vi "Get Conact Check State.vi"(8 "error in (no error)":errorcluster, 10 "Connections  (0: ANY)":u16(ring) items=["ANY", "ALL"], 11 "VISA resource name":refnum<visa-resource-name>="USB0::0x05E6::0x2461::04090176::INSTR") -> (0 "error out":errorcluster, 1 "Guard Check Pass":bool, 2 "Low Check Pass":bool, 3 "VISA resource name out":refnum<visa-resource-name>="USB0::0x05E6::0x2461::04090176::INSTR", 4 "All Contact Checks Pass":bool, 5 "Hi Check Pass":bool)   [LabVIEW 2021, in "Keithley 2450.lvlib"]
doc: "Use this function to check for excessive contact resistance at any of the connections to the device\nunder test (DUT). This function will return an error if Contact Check is not enabled.\n\n<B>The Digitizer Voltage and Digitizer Current functions are only compatible with the 2461.</B>"
uses:
  Keithley 2450.lvlib
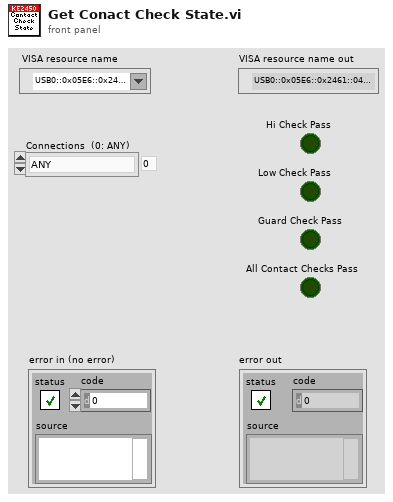
[diagram p1: front panel]
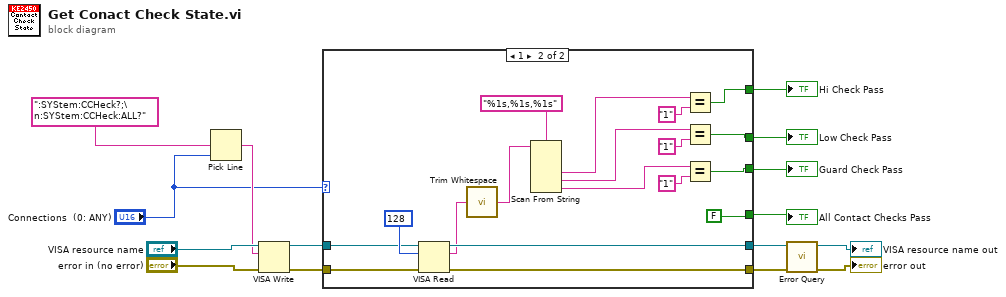
[diagram p0: block diagram]
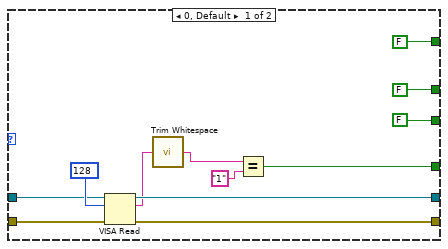
[diagram p2: hidden frame]
diagram:
  n1 = Pick Line(multi-line string=":SYStem:CCHeck?;\n:SYStem:CCHeck:ALL?", line index="Connections  (0: ANY)") -> (output string=w10:string)  [unwired: 1 in]
  n2 = VISA Write(VISA resource name="VISA resource name", write buffer=w10, error in (no error)="error in (no error)") -> (VISA resource name out=w5:refnum<visa-resource-name>, error out=w4:errorcluster)  [unwired: 1 out]
  n3 = case shown="1" "Connections  (0: ANY)" {
    tunnel: [FALSE w43] -> w8
    tunnel: [FALSE w34] -> w7
    tunnel: [FALSE w33] -> w6
    tunnel: w5 -> [w25 w42]
    tunnel: w4 -> [w24 w41]
    tunnel: [w23 w39] -> w3
    tunnel: [w22 w38] -> w2
    tunnel: [w21 FALSE] -> w1
    frame 0, Default {
      n4 = VISA Read(VISA resource name=w25, byte count=u32 128, error in (no error)=w24) -> (VISA resource name out=w23:refnum<visa-resource-name>, read buffer=w16:string, error out=w22:errorcluster)  [unwired: 1 out]
      n5 = call <vilib>:"Trim Whitespace.vi"("string"=w16) -> ("trimmed string"=w17:string)  [unwired: 1 in]
      n6 = Equal?(x=w17, y="1") -> (x = y?=w21:bool)
    }
    frame 1 {
      n7 = VISA Read(VISA resource name=w42, byte count=u32 128, error in (no error)=w41) -> (VISA resource name out=w39:refnum<visa-resource-name>, read buffer=w29:string, error out=w38:errorcluster)  [unwired: 1 out]
      n8 = call <vilib>:"Trim Whitespace.vi"("string"=w29) -> ("trimmed string"=w28:string)  [unwired: 1 in]
      n9 = Scan From String(format string="%1s,%1s,%1s", input string=w28) -> (output 1=w32:string, output 2=w31:string, output 3=w30:string)  [unwired: 5 in, 3 out]
      n10 = Equal?(x=w32, y="1") -> (x = y?=w43:bool)
      n11 = Equal?(x=w31, y="1") -> (x = y?=w34:bool)
      n12 = Equal?(x=w30, y="1") -> (x = y?=w33:bool)
    }
  }
  "Hi Check Pass" <- w8
  "Low Check Pass" <- w7
  "Guard Check Pass" <- w6
  "All Contact Checks Pass" <- w1
  n13 = call "Error Query.vi"("error in (no error)"=w2, "VISA resource name"=w3) -> ("error out"=→"error out":errorcluster, "VISA resource name out"=→"VISA resource name out":refnum<visa-resource-name>)  [unwired: 8 out]
